vi "测试.vi"(5 "I-V扫描":T2, 6 "功能选择":u16(ring) items=["I-V扫描", "脉冲测试", "维持时间"], 7 "脉冲测试":T1, 8 "错误输入":errorcluster, 10 "维持时间":T3, 11 "VISA资源名称":refnum<visa-resource-name>) -> (0 "错误输出":errorcluster, 3 "VISA资源名称输出":refnum<visa-resource-name>)   [LabVIEW 2020]
uses:
  Global variable.vi
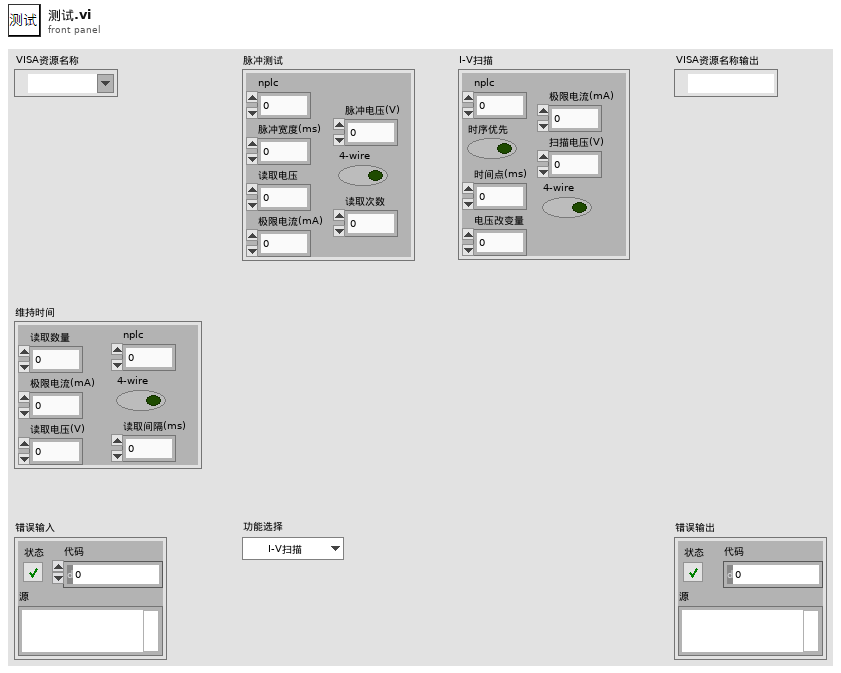
[diagram p1: front panel]
types:
  T1 = cluster{"nplc":dbl, "脉冲宽度(ms)":dbl, "读取电压":dbl, "极限电流(mA)":dbl, "脉冲电压(V)":dbl, "4-wire":bool, "读取次数":dbl}
  T2 = cluster{"nplc":dbl, "时序优先":bool, "时间点(ms)":dbl, "电压改变量":dbl, "极限电流(mA)":dbl, "扫描电压(V)":dbl, "4-wire":bool}
  T3 = cluster{"nplc":dbl, "4-wire":bool, "读取间隔(ms)":dbl, "读取数量":dbl, "极限电流(mA)":dbl, "读取电压(V)":dbl}
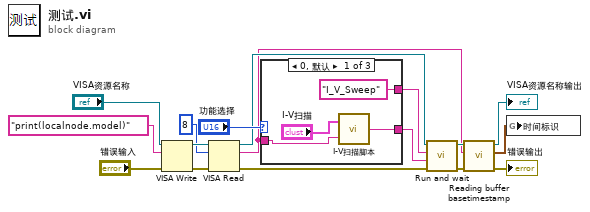
[diagram p0: block diagram]
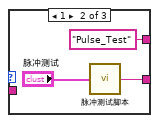
[diagram p2: hidden frame]
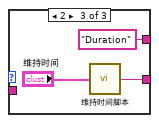
[diagram p3: hidden frame]
diagram:
  n1 = VISA Write(VISA resource name="VISA资源名称", write buffer="print(localnode.model)" ("写入缓冲区"), error in (no error)="错误输入") -> (VISA resource name out=w10:refnum<visa-resource-name>, error out=w9:errorcluster)  [unwired: 1 out]
  n2 = VISA Read(VISA resource name=w10, byte count=u32 8 ("字节总数"), error in (no error)=w9) -> (VISA resource name out=w4:refnum<visa-resource-name>, read buffer=w1:string, error out=w3:errorcluster)  [unwired: 1 out]
  n3 = case shown="0, 默认" "功能选择" {
    tunnel: [w21 w23 w27] -> w13
    tunnel: ["I_V_Sweep" ("Script Name") "Pulse_Test" ("Script Name") "Duration" ("Script Name")] -> w11
    tunnel: w1 -> [w18 _ _]
    frame 0, Default {
      n4 = call "I-V扫描脚本.vi"("仪器型号"=w18, "参数"="I-V扫描") -> ("Script"=w21:string)
    }
    frame 1 {
      n5 = call "脉冲测试脚本.vi"("参数"="脉冲测试") -> ("Script"=w23:string)
    }
    frame 2 {
      n6 = call "维持时间脚本.vi"("参数"="维持时间") -> ("Script"=w27:string)
    }
  }
  n7 = call "Run and wait.vi"("错误输入"=w3, "Script"=w13, "Script Name"=w11, "VISA资源名称"=w4) -> ("错误输出"=w16:errorcluster, "VISA资源名称输出"=w2:refnum<visa-resource-name>)  [unwired: 6 in]
  n8 = call "Reading buffer basetimestamp.vi"("错误输入（无错误）"=w16, "仪器型号"=w1, "VISA资源名称"=w2) -> ("错误输出"=→"错误输出":errorcluster, "时间标识"=w17:timestamp, "VISA资源名称输出"=→"VISA资源名称输出":refnum<visa-resource-name>)  [unwired: 6 in]
  n9 = global write "Global variable.vi" "时间标识"(w17) -> ()
